vi "Action2Trigger.vi"(8 "NewAction?":bool, 9 "Target":dbl, 10 "Enc Initial":dbl, 11 "Current":dbl) -> (0 "Triggered":bool)   [LabVIEW 2017]
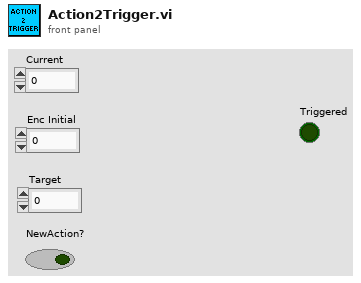
[diagram p1: front panel]
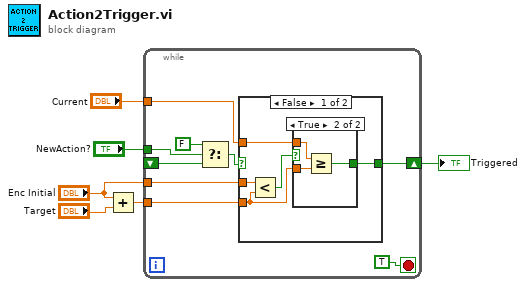
[diagram p0: block diagram]
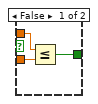
[diagram p2: hidden frame]
diagram:
  n1 = Add(x="Enc Initial", y="Target") -> (x+y=w4:dbl)
  n2 = while {
    tunnel: "Current" -> [w15]
    tunnel: w4 -> [w14]
    tunnel: "NewAction?" -> [w10]
    shift-right: [w11] -> w2
    shift-left: _ -> [w8]
    tunnel: "Enc Initial" -> [w7]
    stop <- TRUE stop-if-true
    n3 = Select(t=FALSE, s=w10, f=w8) -> (s? t:f=w12:bool)
    n4 = case shown="False" w12 {
      selector: w12 -> [_ w27]
      tunnel: w15 -> [w19 _]
      tunnel: w14 -> [w16 _]
      tunnel: [w18 w27] -> w11
      tunnel: w7 -> [w17 _]
      frame False {
        n5 = Less?(x=w17, y=w16) -> (x < y?=w20:bool)
        n6 = case shown="True" w20 {
          tunnel: w16 -> [w23 w24]
          tunnel: w19 -> [w22 w25]
          tunnel: [w21 w26] -> w18
          frame False {
            n7 = Less Or Equal?(x=w22, y=w23) -> (x <= y?=w21:bool)
          }
          frame True {
            n8 = Greater Or Equal?(x=w25, y=w24) -> (x >= y?=w26:bool)
          }
        }
      }
      frame True {
      }
    }
  }
  "Triggered" <- w2
